vi "PDP LeadVoltage= Message.vi"(0 "Lead Voltage":dbl format="%.3f") -> ()   [LabVIEW 2010]
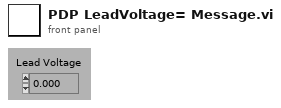
[diagram p1: front panel]
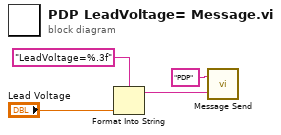
[diagram p0: block diagram]
diagram:
  n1 = Format Into String(format string="LeadVoltage=%.3f" ("Format String"), "Lead Voltage") -> (resulting string=w1:string)  [unwired: 2 in, 1 out]
  n2 = call "Message Send.vi"("Message"=w1, "Destination"="PDP") -> ()
